vi "GUI.vi"() -> ()   [LabVIEW 2019]
uses:
  <vilib>/Instr/_visa.llb/VISA Configure Serial Port (Instr).vi
panel:
  out "DS":dbl
  out "KD":dbl
  out "KI":dbl
  out "KP":dbl
  out "SP":dbl
  in  "Mode":bool
  in  "SP":sgl(slide) min=0 max=1023 scale=0.0..1023.0
  in  "DS":u16(slide) scale=25.0..150.0
  in  "KD":sgl(slide) scale=0.0..10.0
  in  "KI":sgl(slide) scale=0.0..10.0
  in  "KP":sgl(slide) scale=0.0..150.0
  out "O":u16
  out "T":dbl
  out "D":dbl
  out "I":dbl
  out "P":dbl
  out "F":dbl
  out "S":dbl
  in  "Stop Button":bool
  in  "COM Port":refnum<visa-resource-name>
  in  "Save Result":path
  out "Output PID":u16(graph)
  out "Tacho Generator":dbl(knob) scale=0.0..1023.0
  out "SetPoint":dbl(knob) scale=0.0..1023.0
  out "Respon PID":dynamicdata(graph)
  # "ALIM SATRIA FI'I WIJAYA KUSUMA (21/483503/SV/20304)"
  # "KENDALI KECEPATAN MOTOR DC"
  # "ILHAM DWI CAHYO (21/483417/SV/20218)"
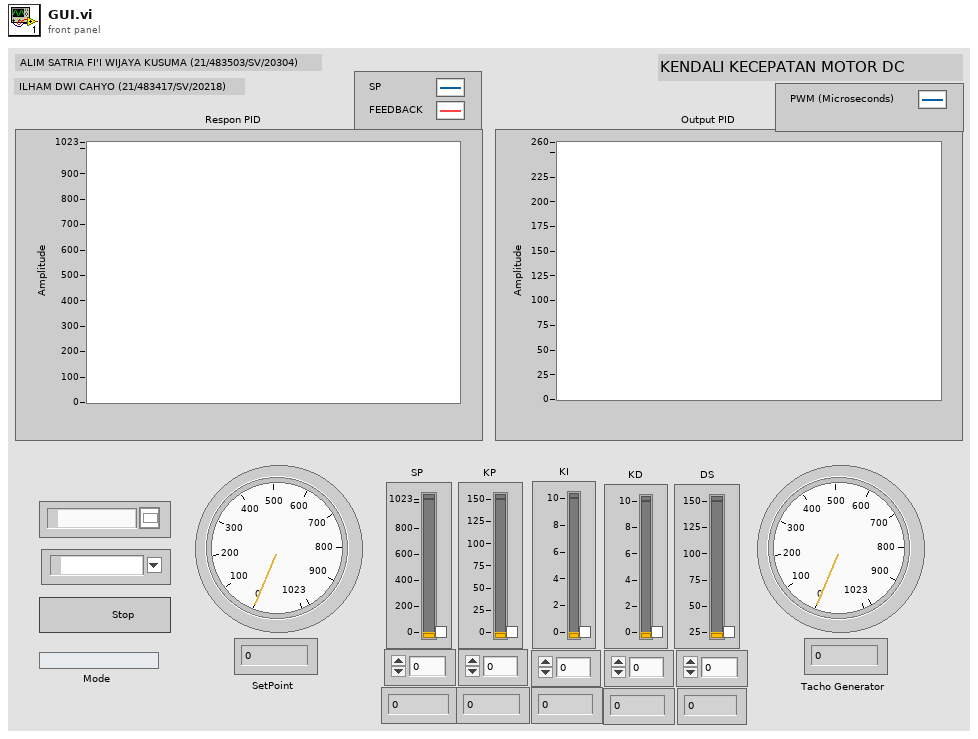
[diagram p1: front panel]
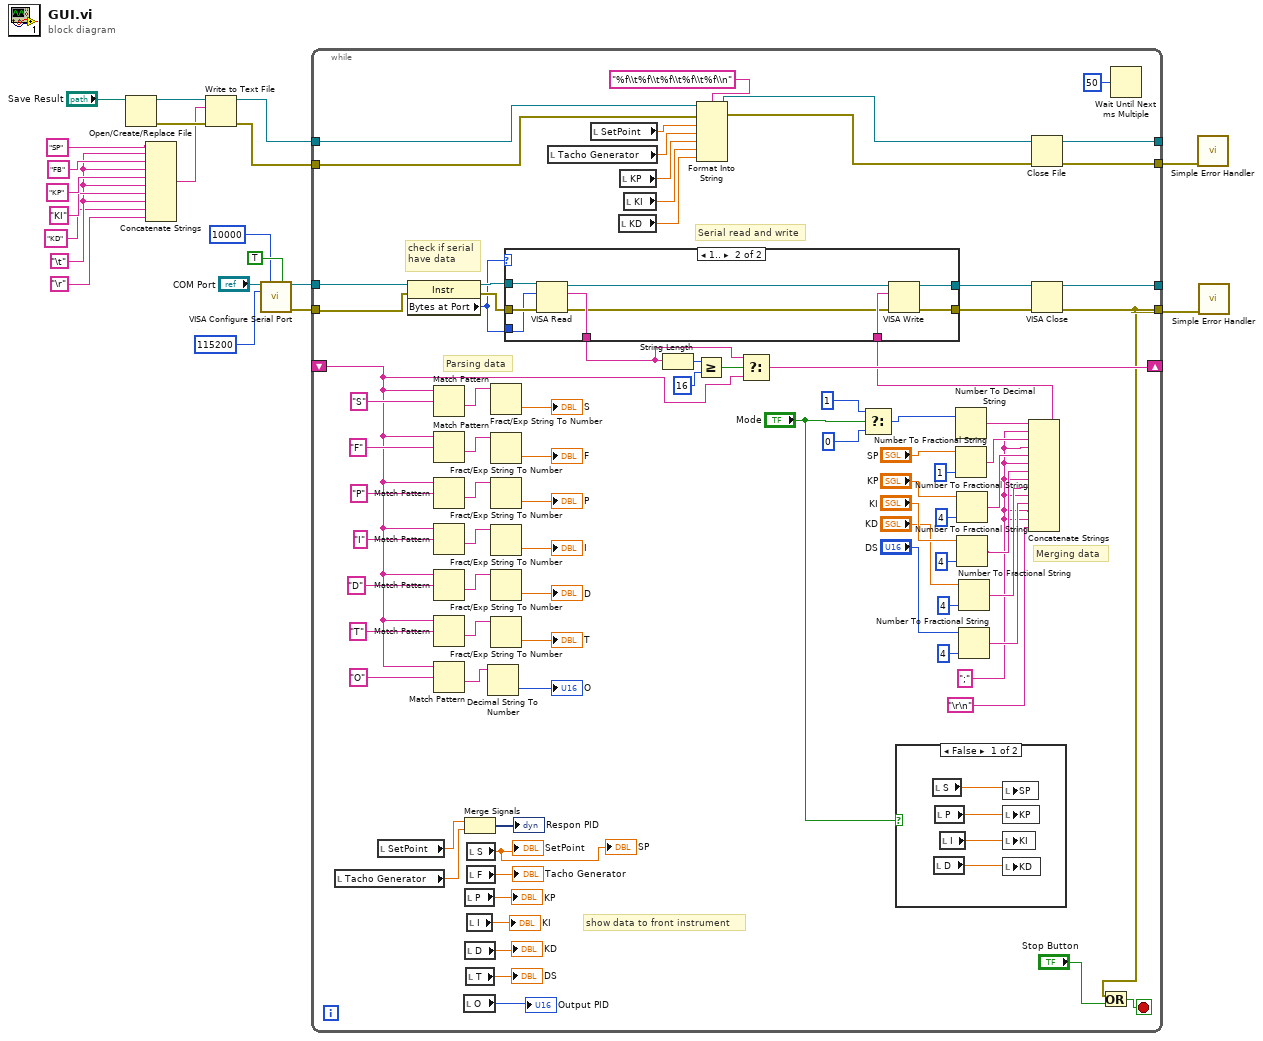
[diagram p0: block diagram]
diagram:
  w8 = "\t"
  n1 = Open/Create/Replace File(file path (use dialog)="Save Result") -> (refnum out=w18:refnum<file>, error out=w19:errorcluster)  [unwired: 5 in, 1 out]
  n2 = Concatenate Strings("SP", w8, "FB" ("string"), w8, "KP" ("string"), w8, "KI" ("string"), w8, "KD" ("string"), "\r") -> (w13:string)
  n3 = Write to Text File(file (use dialog)=w18, text=w13, error in=w19) -> (refnum out=w17:refnum<file>, error out=w16:errorcluster)  [unwired: 1 in, 1 out]
  n4 = call-poly "VISA Configure Serial Port"("VISA resource name"="COM Port", "timeout (10sec)"=u32 10000, "Enable Termination\nChar (T)"=TRUE ("Enable Termination\nChar (T)"), "baud rate (9600)"=u32 115200) -> ("VISA resource name out"=w25:refnum<visa-resource-name>, "error out"=w24:errorcluster)  [unwired: 10 in]
  n5 = while {
    tunnel: w25 -> [w54]
    tunnel: w24 -> [w53]
    tunnel: [w51] -> w23
    tunnel: [w50] -> w22
    tunnel: w17 -> [w80]
    tunnel: w16 -> [w79]
    tunnel: [w78] -> w15
    tunnel: [w77] -> w14
    shift-right: [w70] -> _
    shift-left: _ -> [w69]
    stop <- w105 stop-if-true
    w29 = ";"
    # "show data to front instrument"
    # "check if serial\nhave data"
    # "Serial read and write"
    # "Merging data"
    # "Parsing data"
    n6 = local read "Tacho Generator"() -> (w82:dbl)
    n7 = local read "SetPoint"() -> (w83:dbl)
    n8 = property class="Instr"(reference=w54, error in=w53) -> (reference out=w67:refnum<visa-resource-name>, error out=w66:errorcluster, "Bytes at Port"=w30:u32)
    n9 = Match Pattern(string=w69, regular expression="S") -> (after substring=w96:string)  [unwired: 1 in, 3 out]
    n10 = Match Pattern(string=w69, regular expression="F") -> (after substring=w95:string)  [unwired: 1 in, 3 out]
    n11 = Match Pattern(string=w69, regular expression="P") -> (after substring=w94:string)  [unwired: 1 in, 3 out]
    n12 = Match Pattern(string=w69, regular expression="I") -> (after substring=w93:string)  [unwired: 1 in, 3 out]
    n13 = Match Pattern(string=w69, regular expression="D") -> (after substring=w92:string)  [unwired: 1 in, 3 out]
    n14 = Match Pattern(string=w69, regular expression="T") -> (after substring=w91:string)  [unwired: 1 in, 3 out]
    n15 = Match Pattern(string=w69, regular expression="O") -> (after substring=w31:string)  [unwired: 1 in, 3 out]
    n16 = local read "O"() -> (→"Output PID":u16)
    n17 = Merge Signals(w83, w82) -> (→"Respon PID":dynamicdata)
    n18 = local read "P"() -> (→"KP":dbl)
    n19 = local read "D"() -> (→"KD":dbl)
    n20 = local read "T"() -> (→"DS":dbl)
    n21 = local read "S"() -> (→"SetPoint" →"SP":dbl)
    n22 = local read "F"() -> (→"Tacho Generator":dbl)
    n23 = local read "I"() -> (→"KI":dbl)
    n24 = Decimal String To Number(string=w31) -> (number=→"O":i32)  [unwired: 2 in, 1 out]
    n25 = Fract/Exp String To Number(string=w96) -> (number=→"S":dbl)  [unwired: 3 in, 1 out]
    n26 = Fract/Exp String To Number(string=w95) -> (number=→"F":dbl)  [unwired: 3 in, 1 out]
    n27 = Fract/Exp String To Number(string=w94) -> (number=→"P":dbl)  [unwired: 3 in, 1 out]
    n28 = Fract/Exp String To Number(string=w93) -> (number=→"I":dbl)  [unwired: 3 in, 1 out]
    n29 = Fract/Exp String To Number(string=w92) -> (number=→"D":dbl)  [unwired: 3 in, 1 out]
    n30 = Fract/Exp String To Number(string=w91) -> (number=→"T":dbl)  [unwired: 3 in, 1 out]
    n31 = local read "Tacho Generator"() -> (w75:dbl)
    n32 = local read "SetPoint"() -> (w76:dbl)
    n33 = local read "KD"() -> (w55:dbl)
    n34 = local read "KP"() -> (w57:dbl)
    n35 = local read "KI"() -> (w56:dbl)
    n36 = Format Into String(format string="%f\\t%f\\t%f\\t%f\\t%f\\n", initial string=w80, error in=w79, w76, w75, w57, w56, w55) -> (resulting string=w78:refnum<file>, error out=w77:errorcluster)
    n37 = Select(t=u8 1, s="Mode", f=u8 0) -> (s? t:f=w40:u8)
    n38 = case shown="False" "Mode" {
      frame False {
        n39 = local read "S"() -> (w106:dbl)
        n40 = local read "D"() -> (w107:dbl)
        n41 = local read "P"() -> (w109:dbl)
        n42 = local read "I"() -> (w108:dbl)
        n43 = local write "SP"(w106) -> ()
        n44 = local write "KP"(w109) -> ()
        n45 = local write "KI"(w108) -> ()
        n46 = local write "KD"(w107) -> ()
      }
      frame True {
      }
    }
    n47 = Number To Decimal String(number=w40) -> (decimal integer string=w39:string)  [unwired: 1 in]
    n48 = Number To Fractional String(number="SP", precision (6)=i16 1) -> (F-format string=w38:string)  [unwired: 2 in]
    n49 = Number To Fractional String(number="KP", precision (6)=i16 4) -> (F-format string=w37:string)  [unwired: 2 in]
    n50 = Number To Fractional String(number="KI", precision (6)=i16 4) -> (F-format string=w36:string)  [unwired: 2 in]
    n51 = Number To Fractional String(number="KD", precision (6)=i16 4) -> (F-format string=w35:string)  [unwired: 2 in]
    n52 = Number To Fractional String(number="DS", precision (6)=i16 4) -> (F-format string=w34:string)  [unwired: 2 in]
    n53 = Concatenate Strings(w39, w29, w38, w29, w37, w29, w36, w29, w35, w29, w34, w29, w29, "\r\n") -> (w33:string)
    n54 = case shown="1.." w30 {
      tunnel: [_ w120] -> w68
      tunnel: w67 -> [w111 w119]
      tunnel: w66 -> [w110 w118]
      tunnel: [w111 w117] -> w51
      tunnel: [w110 w116] -> w50
      tunnel: w33 -> [_ w115]
      tunnel: w30 -> [_ w112]
      frame 0, Default {
      }
      frame 1.. {
        n55 = VISA Read(VISA resource name=w119, byte count=w112, error in (no error)=w118) -> (VISA resource name out=w114:refnum<visa-resource-name>, read buffer=w120:string, error out=w113:errorcluster)  [unwired: 1 out]
        n56 = VISA Write(VISA resource name=w114, write buffer=w115, error in (no error)=w113) -> (VISA resource name out=w117:refnum<visa-resource-name>, error out=w116:errorcluster)  [unwired: 1 out]
      }
    }
    n57 = String Length(string=w68) -> (length=w73:i32)
    n58 = Greater Or Equal?(x=w73, y=16) -> (x >= y?=w71:bool)
    n59 = Select(t=w68, s=w71, f=w69) -> (s? t:f=w70:string)
    n60 = Or(x=w50, y="Stop Button") -> (x .or. y?=w105:bool)
    n61 = Wait Until Next ms Multiple(millisecond multiple=u32 50) -> ()  [unwired: 1 out]
  }
  n62 = Close File(refnum=w15, error in=w14) -> (error out=w5:errorcluster)  [unwired: 1 out]
  n63 = VISA Close(VISA resource name=w23, error in (no error)=w22) -> (error out=w4:errorcluster)
  n64 = call <vilib>:"Simple Error Handler.vi"("error in (no error)"=w5) -> ()  [unwired: 4 in, 5 out]
  n65 = call <vilib>:"Simple Error Handler.vi"("error in (no error)"=w4) -> ()  [unwired: 4 in, 5 out]
